vi "provide_OME_data.vi"(6 "image ID":string, 8 "error in (no error)":errorcluster, 9 "structuredAttribute string in":string, 10 "OME element in":refnum<class "XMLElement.lvclass">, 11 "LightSourceDL090903Laser in":refnum<class "LightSourceDL090903Laser.lvclass">) -> (0 "error out":errorcluster, 1 "structuredAttribute string out":string, 2 "OME element out":refnum<class "XMLElement.lvclass">, 3 "LightSourceDL090903Laser out":refnum<class "LightSourceDL090903Laser.lvclass">)   [LabVIEW 2010, in "LightSourceDL090903Laser.lvclass"]
uses:
  LightSourceDL090903Laser.lvclass
  common/classes/XMLElement/XMLElement/XMLElement.lvclass
  GenericLightSource/GenericLightSource/GenericLightSource.lvclass
  LightSourceDL090903Laser.lvclass/LightSourceDL090903Laser.ctl
  Instrument/GenericInstrument/GenericInstrument/GenericInstrument.lvclass
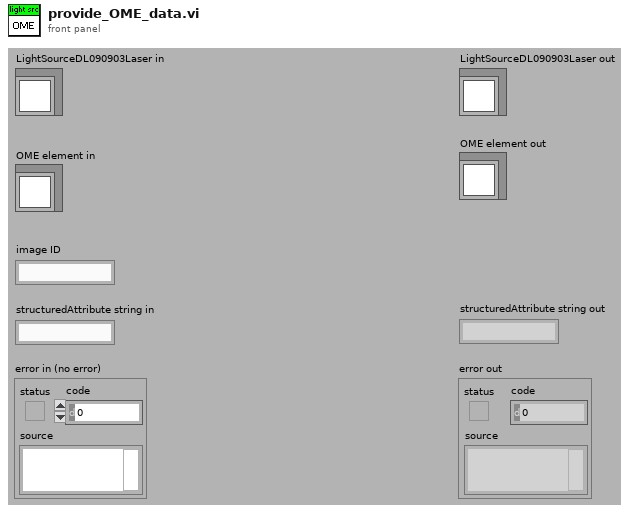
[diagram p1: front panel]
types:
  T1 = typedef "LightSourceDL090903Laser.lvclass/type_enum.ctl" = enum16{"Excimer", "Gas", "MetalVapor", "SolidState", "Dye", "Semiconductor", "FreeElectron", "Unknown"}
  T2 = typedef "LightSourceDL090903Laser.lvclass/laser_medium_enum.ctl" = enum16{"Cu", "Ag", "ArFl", "ArCl", "KrFl", "XeFl", "XeCl", "XeBr", "N", "Ar", "Kr", "Xe", "HeNe", "HeCd", "CO", "CO2", "H2O", "HFl", "NdGlass", "NdYAG", "ErGlass", "ErYAG", "HoYLF", "HoYAG", "Ruby", "TiSapphire", "Alexandrite", "Rhodamine6G", "CoumarineC30", "GaAs", "GaAlAs", "EMinus", "Unknown"}
  T3 = typedef "LightSourceDL090903Laser.lvclass/pulse_enum.ctl" = enum16{"CW", "Single", "QSwitched", "Repetitive", "ModeLocked"}
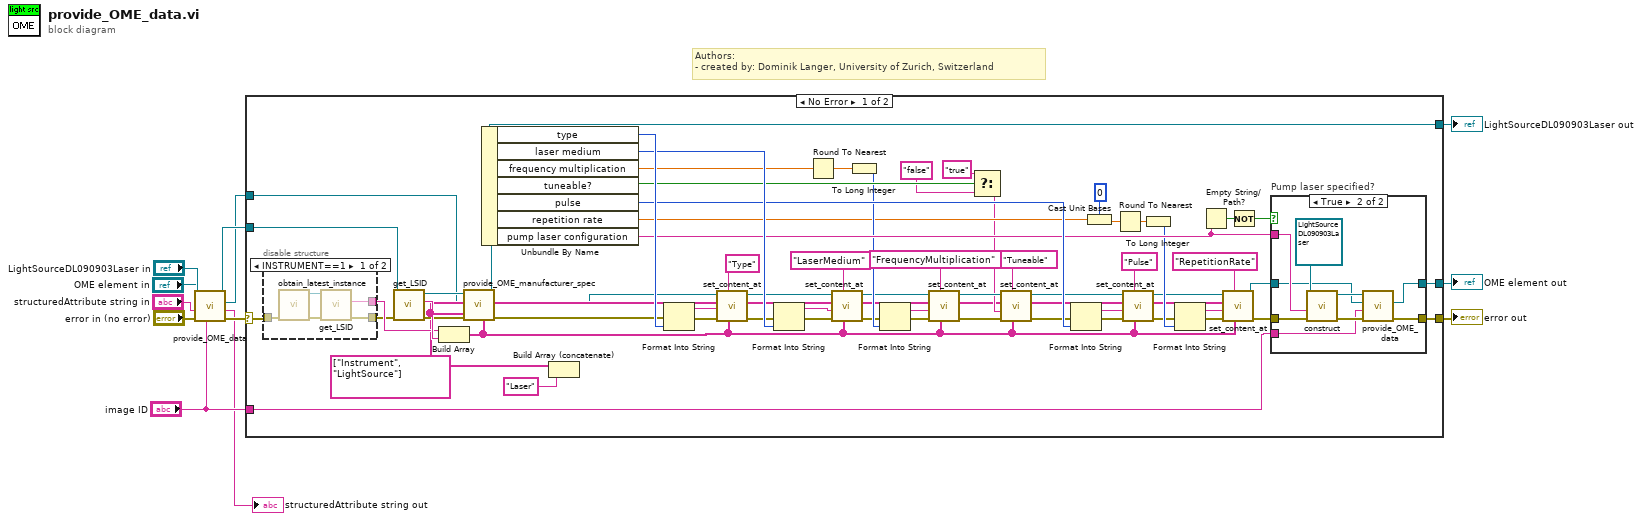
[diagram p0: block diagram]
diagram:
  # "Authors: \n- created by: Dominik Langer, University of Zurich, Switzerland"
  n1 = call-parent "provide_OME_data.vi"("image ID"="image ID", "error in (no error)"="error in (no error)", "structuredAttribute string in"="structuredAttribute string in", "OME element in"="OME element in", "GenericPlugin in"="LightSourceDL090903Laser in") -> ("error out"=w10:errorcluster, "structuredAttribute string out"=→"structuredAttribute string out":string, "OME element out"=w6:refnum<class "XMLElement.lvclass">, "GenericPlugin out"=w9:refnum<class "LightSourceDL090903Laser.lvclass">)  [unwired: 3 in]
  n2 = case shown="No Error" w10 {
    selector: w10 -> [w53 w95]
    tunnel: w9 -> [w52 w94]
    tunnel: [w69 w95] -> w8
    tunnel: [w18 w94] -> w7
    tunnel: w6 -> [w14 w93]
    tunnel: [w70 w93] -> w4
    tunnel: "image ID" -> [w35 _]
    frame No Error {
      w15 = string[] ["Instrument", "LightSource"]
      n3 = disable-structure shown="INSTRUMENT==1" {
        disable-tunnel: w53 -> [w78 w81]
        disable-tunnel: [w77 w81] -> w54
        disable-tunnel: [w76 _] -> w55
        frame condition #0 {
          n4 = call "obtain_latest_instance.vi"("error in (no error)"=w78) -> ("error out"=w79:errorcluster, "microscope"=w80:refnum<class "GenericInstrument.lvclass">)  [unwired: 9 in]
          n5 = call-dynamic "get_LSID.vi"("error in (no error)"=w79, "GenericPlugin in"=w80) -> ("error out"=w77:errorcluster, "LSID (string)"=w76:string)  [unwired: 6 in, 2 out]
        }
        frame condition #1 (active) {
        }
      }
      n6 = call-dynamic "get_LSID.vi"("error in (no error)"=w54, "GenericPlugin in"=w52) -> ("error out"=w20:errorcluster, "LSID (string)"=w56:string, "GenericPlugin out"=w21:refnum<class "LightSourceDL090903Laser.lvclass">)  [unwired: 6 in, 1 out]
      n7 = Build Array(w55, w56) -> (w17:string[])
      n8 = call-dynamic "provide_OME_manufacturer_spec.vi"("id chain"=w17, "key chain"=w15, "error in (no error)"=w20, "XMLElement in"=w14, "GenericPlugin in"=w21) -> ("error out"=w19:errorcluster, "XMLElement out"=w13:refnum<class "XMLElement.lvclass">, "GenericPlugin out"=w18:refnum<class "LightSourceDL090903Laser.lvclass">)  [unwired: 4 in]
      n9 = Unbundle By Name(w18) -> ("type"=w75:T1, "laser medium"=w74:T2, "frequency multiplication"=w63:dbl, "tuneable?"=w67:bool, "pulse"=w73:T3, "repetition rate"=w58:dbl[unit], "pump laser configuration"=w68:string)
      n10 = Build Array (concatenate)(w15, "Laser") -> ()  [unwired: 1 out]
      n11 = Format Into String(error in=w19, w75) -> (resulting string=w33:string, error out=w51:errorcluster)  [unwired: 2 in]
      n12 = call "set_content_at.vi"("id chain"=w17, "attribute name"="Type" ("String"), "error in (no error)"=w51, "content"=w33, "key chain"=w15, "Element in"=w13) -> ("error out"=w50:errorcluster, "Element out"=w48:refnum<class "XMLElement.lvclass">)  [unwired: 4 in]
      n13 = Format Into String(error in=w50, w74) -> (resulting string=w31:string, error out=w49:errorcluster)  [unwired: 2 in]
      n14 = Round To Nearest(number=w63) -> (nearest integer value=w64:dbl)
      n15 = call "set_content_at.vi"("id chain"=w17, "attribute name"="LaserMedium" ("String"), "error in (no error)"=w49, "content"=w31, "key chain"=w15, "Element in"=w48) -> ("error out"=w47:errorcluster, "Element out"=w45:refnum<class "XMLElement.lvclass">)  [unwired: 4 in]
      n16 = To Long Integer(number=w64) -> (32bit integer=w62:i32)
      n17 = Format Into String(error in=w47, w62) -> (resulting string=w28:string, error out=w46:errorcluster)  [unwired: 2 in]
      n18 = call "set_content_at.vi"("id chain"=w17, "attribute name"="FrequencyMultiplication" ("String"), "error in (no error)"=w46, "content"=w28, "key chain"=w15, "Element in"=w45) -> ("error out"=w44:errorcluster, "Element out"=w43:refnum<class "XMLElement.lvclass">)  [unwired: 4 in]
      n19 = Select(t="true", s=w67, f="false") -> (s? t:f=w26:string)
      n20 = call "set_content_at.vi"("id chain"=w17, "attribute name"="Tuneable" ("String"), "error in (no error)"=w44, "content"=w26, "key chain"=w15, "Element in"=w43) -> ("error out"=w42:errorcluster, "Element out"=w41:refnum<class "XMLElement.lvclass">)  [unwired: 4 in]
      n21 = Format Into String(error in=w42, w73) -> (resulting string=w25:string, error out=w34:errorcluster)  [unwired: 2 in]
      n22 = Cast Unit Bases(0:w58, 1:0) -> (2:w60:dbl)
      n23 = Round To Nearest(number=w60) -> (nearest integer value=w61:dbl)
      n24 = call "set_content_at.vi"("id chain"=w17, "attribute name"="Pulse" ("String"), "error in (no error)"=w34, "content"=w25, "key chain"=w15, "Element in"=w41) -> ("error out"=w40:errorcluster, "Element out"=w38:refnum<class "XMLElement.lvclass">)  [unwired: 4 in]
      n25 = To Long Integer(number=w61) -> (32bit integer=w57:i32)
      n26 = Format Into String(error in=w40, w57) -> (resulting string=w22:string, error out=w39:errorcluster)  [unwired: 2 in]
      n27 = Empty String/Path?(string/path=w68) -> (empty?=w72:bool)
      n28 = call "set_content_at.vi"("id chain"=w17, "attribute name"="RepetitionRate" ("String"), "error in (no error)"=w39, "content"=w22, "key chain"=w15, "Element in"=w38) -> ("error out"=w37:errorcluster, "Element out"=w36:refnum<class "XMLElement.lvclass">)  [unwired: 4 in]
      n29 = Not(x=w72) -> (.not. x?=w71:bool)
      n30 = case "Pump laser specified?" shown="True" w71 {
        tunnel: w37 -> [w82 w92]
        tunnel: w36 -> [w83 w86]
        tunnel: [w83 w85] -> w70
        tunnel: [w82 w88] -> w69
        tunnel: w68 -> [_ w90]
        tunnel: w35 -> [_ w84]
        frame False {
        }
        frame True {
          n31 = call-dynamic "construct.vi"("error in (no error)"=w92, "configuration name"=w90, "GenericPlugin in"=refnum<class "LightSourceDL090903Laser.lvclass"> refnum ("LightSourceDL090903Laser.lvclass")) -> ("error out"=w89:errorcluster, "GenericPlugin out"=w87:refnum<class "LightSourceDL090903Laser.lvclass">)  [unwired: 7 in]
          n32 = call-dynamic "provide_OME_data.vi"("error in (no error)"=w89, "structuredAttribute string in"=w84, "OME element in"=w86, "LightSourceDL090903Laser in"=w87) -> ("error out"=w88:errorcluster, "OME element out"=w85:refnum<class "XMLElement.lvclass">)  [unwired: 4 in, 2 out]
        }
      }
    }
    frame Error {
    }
  }
  "error out" <- w8
  "LightSourceDL090903Laser out" <- w7
  "OME element out" <- w4
